vi "AG_PertApp.vi"() -> ()   [LabVIEW 2018]
doc: "The myRIO Project template acquires acceleration data from the onboard accelerometer and displays the changes of acceleration values in a waveform chart."
uses:
  <vilib>/Platform/TimedLoop/XDataNode/timing_clust.ctl
  <vilib>/Platform/TimedLoop/XDataNode/nitl_modes.ctl
  <vilib>/Platform/TimedLoop/XDataNode/wakeup.ctl
  <vilib>/Analysis/baseanly.llb/Mean (DBL).vi
  <vilib>/Analysis/1siggen.llb/Riffle Array (DBL).vi
  <vilib>/platform/TimedLoop/XDataNode/XDataNode.xnode
  <vilib>/Platform/TimedLoop/XDataNode/XDNodeRunTimeDep.lvlib
  <vilib>/Analysis/NI_AALBase.lvlib
  <vilib>/express/express signal manip/GetorSetDDTAttributes/Set DDT Attributes/Set DDT Properties.xnode
  <vilib>/express/express shared/transition.llb/Dynamic To Waveform Array.vi
  <vilib>/express/express signal manip/GetorSetDDTAttributes/Set DDT Attributes/SetT0.vi
  <vilib>/express/express shared/transition.llb/Waveform Array To Dynamic.vi
panel:
  in  "device name":tag="Dev1"
  in  "Developer Mode":bool
  out "Packet Array\nString":string
  out "Pert?":dbl
  in  "file path (use dialog)":path
  in  "Rest Steps\nCounter":bool
  in  "?":bool
  in  "Remote Port":u16=4000
  in  "IP Address":string="127.0.0.1"
  in  "Export Log Pathfile":path=path "test.xlsx" caption="Filename"
  in  "Perturbation Parameter\nArray Filepath":path=path "test.lvm" caption="Filename"
  in  "Perturbation \nSetting":enum32{"Predetermine", "Random", "Manual"}(radio)=enum."Manual"
  out "Step\nArray":dbl[](array[numeric])
  out "Perturbation\nArray":dbl[](array[numeric])
  in  "OK Button":bool
  out "Trial Number":dbl=1.0
  in  "Speed Parameter":enum32{"0.7 m/s Settings", "1.0 m/s Settings"}(radio)
  out "Packet Boolean":u32
  out "Packet \nArray":u8[][](array[numeric])
  out "Left vGRF (Filtered)":dynamicdata(graph)
  out "Step Counter":dbl
  in  "?":bool
  in  "GRF \nThreshold":dbl=30.0
  in  "Stance Fraction\nTrip":dbl=0.4
  out "Perturbation\nDelay Onset":dbl
  in  "LHS - Slip":bool
  in  "LHS Trip":bool
  in  "RHS - Slip":bool
  out "RHS?":bool
  out "TM Accel/\nDecel":dbl
  in  "RHS - Trip":bool
  out "HS Delay":dbl
  out "LHS?":bool
  in  "Slip/Trip \nTimer":dbl=0.2
  in  "Right Trip":bool
  in  "Left Trip":bool
  in  "Right Slip":bool
  in  "Left Slip":bool
  out "Right vGRF":dbl
  out "Left vGRF":dbl
  out "R-Stance\nMean":dbl format="%0.2f"
  out "LTO":dbl[](array[numeric])
  out "L-Stance Time":dbl[](array[numeric])
  out "LHS":dbl[](array[numeric])
  out "L-Stance\nMean":dbl format="%0.2f"
  out "R-Stance Time":dbl[](array[numeric])
  out "RTO":dbl[](array[numeric])
  out "RHS":dbl[](array[numeric])
  out "Elapsed Time (s)":dbl
  out "Right vGRF (Filtered)":dynamicdata(graph)
  in  "Stance Fraction\nSlip":dbl=0.4
  in  "Treadmill Control":bool
  in  "Treadmill Stop":bool
  in  "Belt Accel":dbl
  in  "Trip Speed":dbl
  in  "Slip Speed":dbl=2.0
  in  "Decelerate":dbl=10.0
  in  "Accelerate":dbl=10.0
  in  "Belt Speed":dbl(slide) min=0.0 step=0.1 scale=0.0..10.0
  out "TM Connection":errorcluster
  in  "Stop":bool
  # "Treadmill Control Protocol: READ FIRST\n\nBEFORE RUNNING VI\n1. Set \"Pertubration Parameters\" to either \"Predetermine\",\"Random\", or \"Manual\"\n\n1a. If set to \"Predetermine\", go into sub-VI and input all numbers into the \nPerturbation Array\" and \"Step Array\" in the \"Initialize\" part of the flat sequence\n\n2. Ensure all parameters are set to desired values. \n\n3. Optional: Input Filepath for text file \n\nSTART VI\n\n4. Press \"START\" on Treadmill Control Button. This will prevent the belt from accelerating more than 0.2 m/s^2. The treadmill will not start moving at this point\n\n5. Set Belt Speed to desired speed. \n\n5. Press \"Rest Step Counter\" to reset step counter once belt is up to speed\n\n6. DO NOT TURN OFF \"START\" TREADMILL CONTROL BUTTON UNTIL DESIRED SPEED IS MET! The treadmill will accelerate/decelerate at 10m/s^2 when the button is off\n\n7. Turn off \"START\"\"Treadmill Control Button once the desired speed is reached.\n\n8. Allow for a minimum of 5-steps per side to calculate average stance time for both feet\n\n9. Once average stance is calculated initiate a slip/trip my pressing Slip/Trip button for the corresponding side\n\n10. Allow for a minumum of 5-steps after perturbation to calculate average stance time again\n\n11. Continue steps 8-10 until all slips/trips have been performed.\n\n12. To slow the treadmill down, press the Treadmill \"STOP: button. This will decelerate the treadmill to 0 m/s at a rate of 0.2 m/s^2. \n\nIMPORTANT: If the belt speed needs to be changed after the initial speed is set, the \"START\" on theTreadmill Control Button must be enabled. If it is not enabled, the belt will accelerate at 10.0 m/s^2\n\nUse Left and Right Zero if needed"
  # "Perturbations"
  # "Perturabtion Paremeters"
  # "Developer Mode\n\nUse developer mode to test slipping protocol without vGRF data. \n\n1. Turn on \"Developer Mode\" button\n\n2. Press perturbation button\n\n3. Press corresponding developer button to emulate a heel strike"
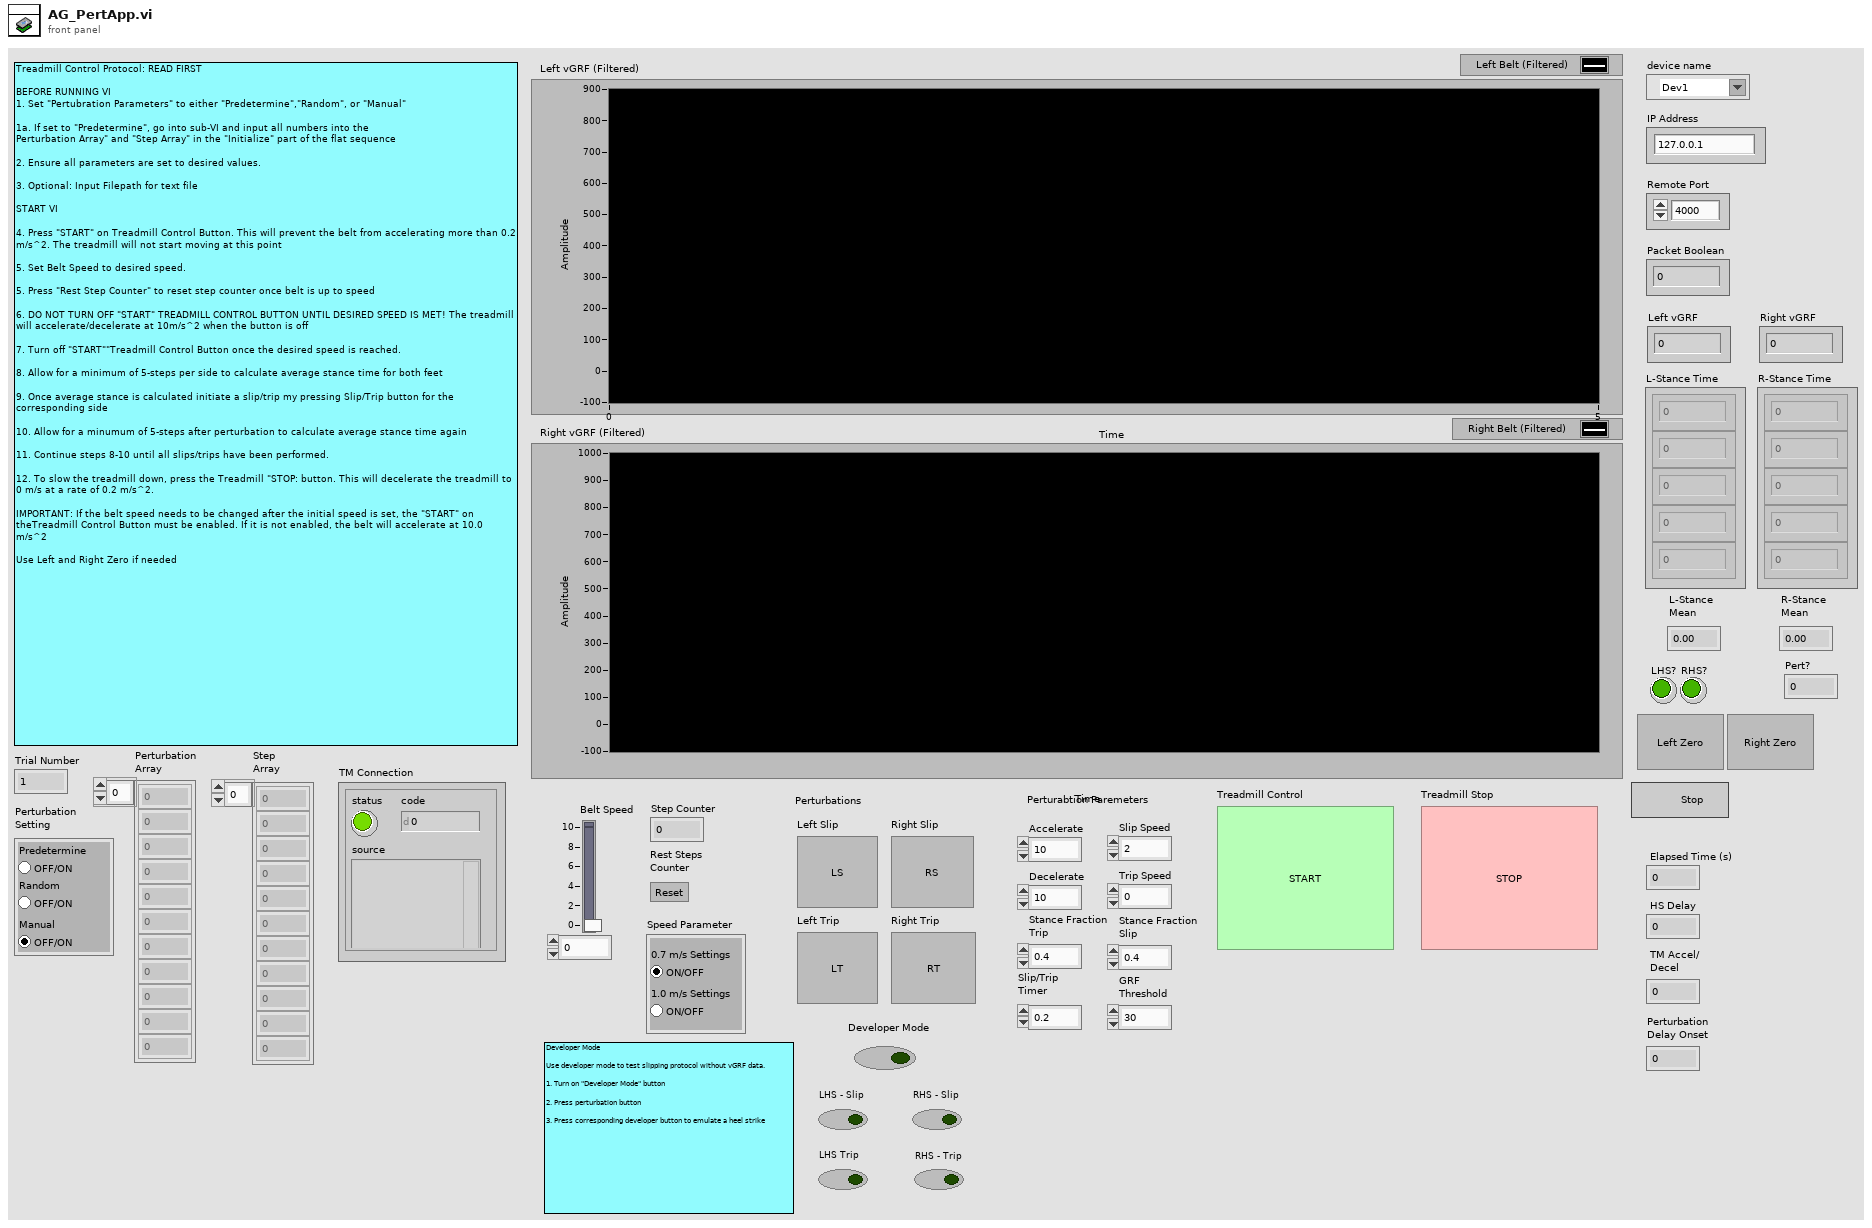
[diagram p1: front panel]
types:
  T1 = enum16{"open", "replace", "create", "open or create", "replace or create", "replace or create with confirmation"}
  T2 = enum16{"big-endian, network order", "native, host order", "little-endian"}
  T3 = typedef "XDNodeRunTimeDep.lvlib/timing_clust.ctl" = cluster{"Expected End [f-1]":u64, "Actual End [f-1]":u64, "Finished Late? [f-1]":bool, "Expected End [i-1]":u64, "Actual End [i-1]":u64, "Finished Late? [i-1]":bool, "Expected Start [i]":u64, "Actual Start [i]":u64, "Expected Start [f]":u64, "Actual Start [f]":u64, "Source Name":string, "Structure Name":string, "Period":i64, "Deadline":i64, "Offset":i64, "Start":i64, "Priority":i32, "Timeout":i32, "Mode":T4, "Wakeup Reason":T5, "Error":errorcluster, "Source Type":string, "Secondary Source Type":string, "Global End Time":u64, "Global Start Time":u64, "Frame Duration":u64, "Iteration Duration":u64, "Assigned CPU":i32, "I/O Scan Engine Mode":u32}
  T4 = typedef "XDNodeRunTimeDep.lvlib/nitl_modes.ctl" = enum32{"No Change", "Process missed periods, maintain original phase", "Discard missed periods, maintain original phase", "Process missed periods, ignore original phase", "Discard missed periods, ignore original phase"}
  T5 = typedef "XDNodeRunTimeDep.lvlib/wakeup.ctl" = enum32{"Normal", "Aborted", "Asynchronous wakeup", "Timing source error", "Timed loop error", "Timeout"}
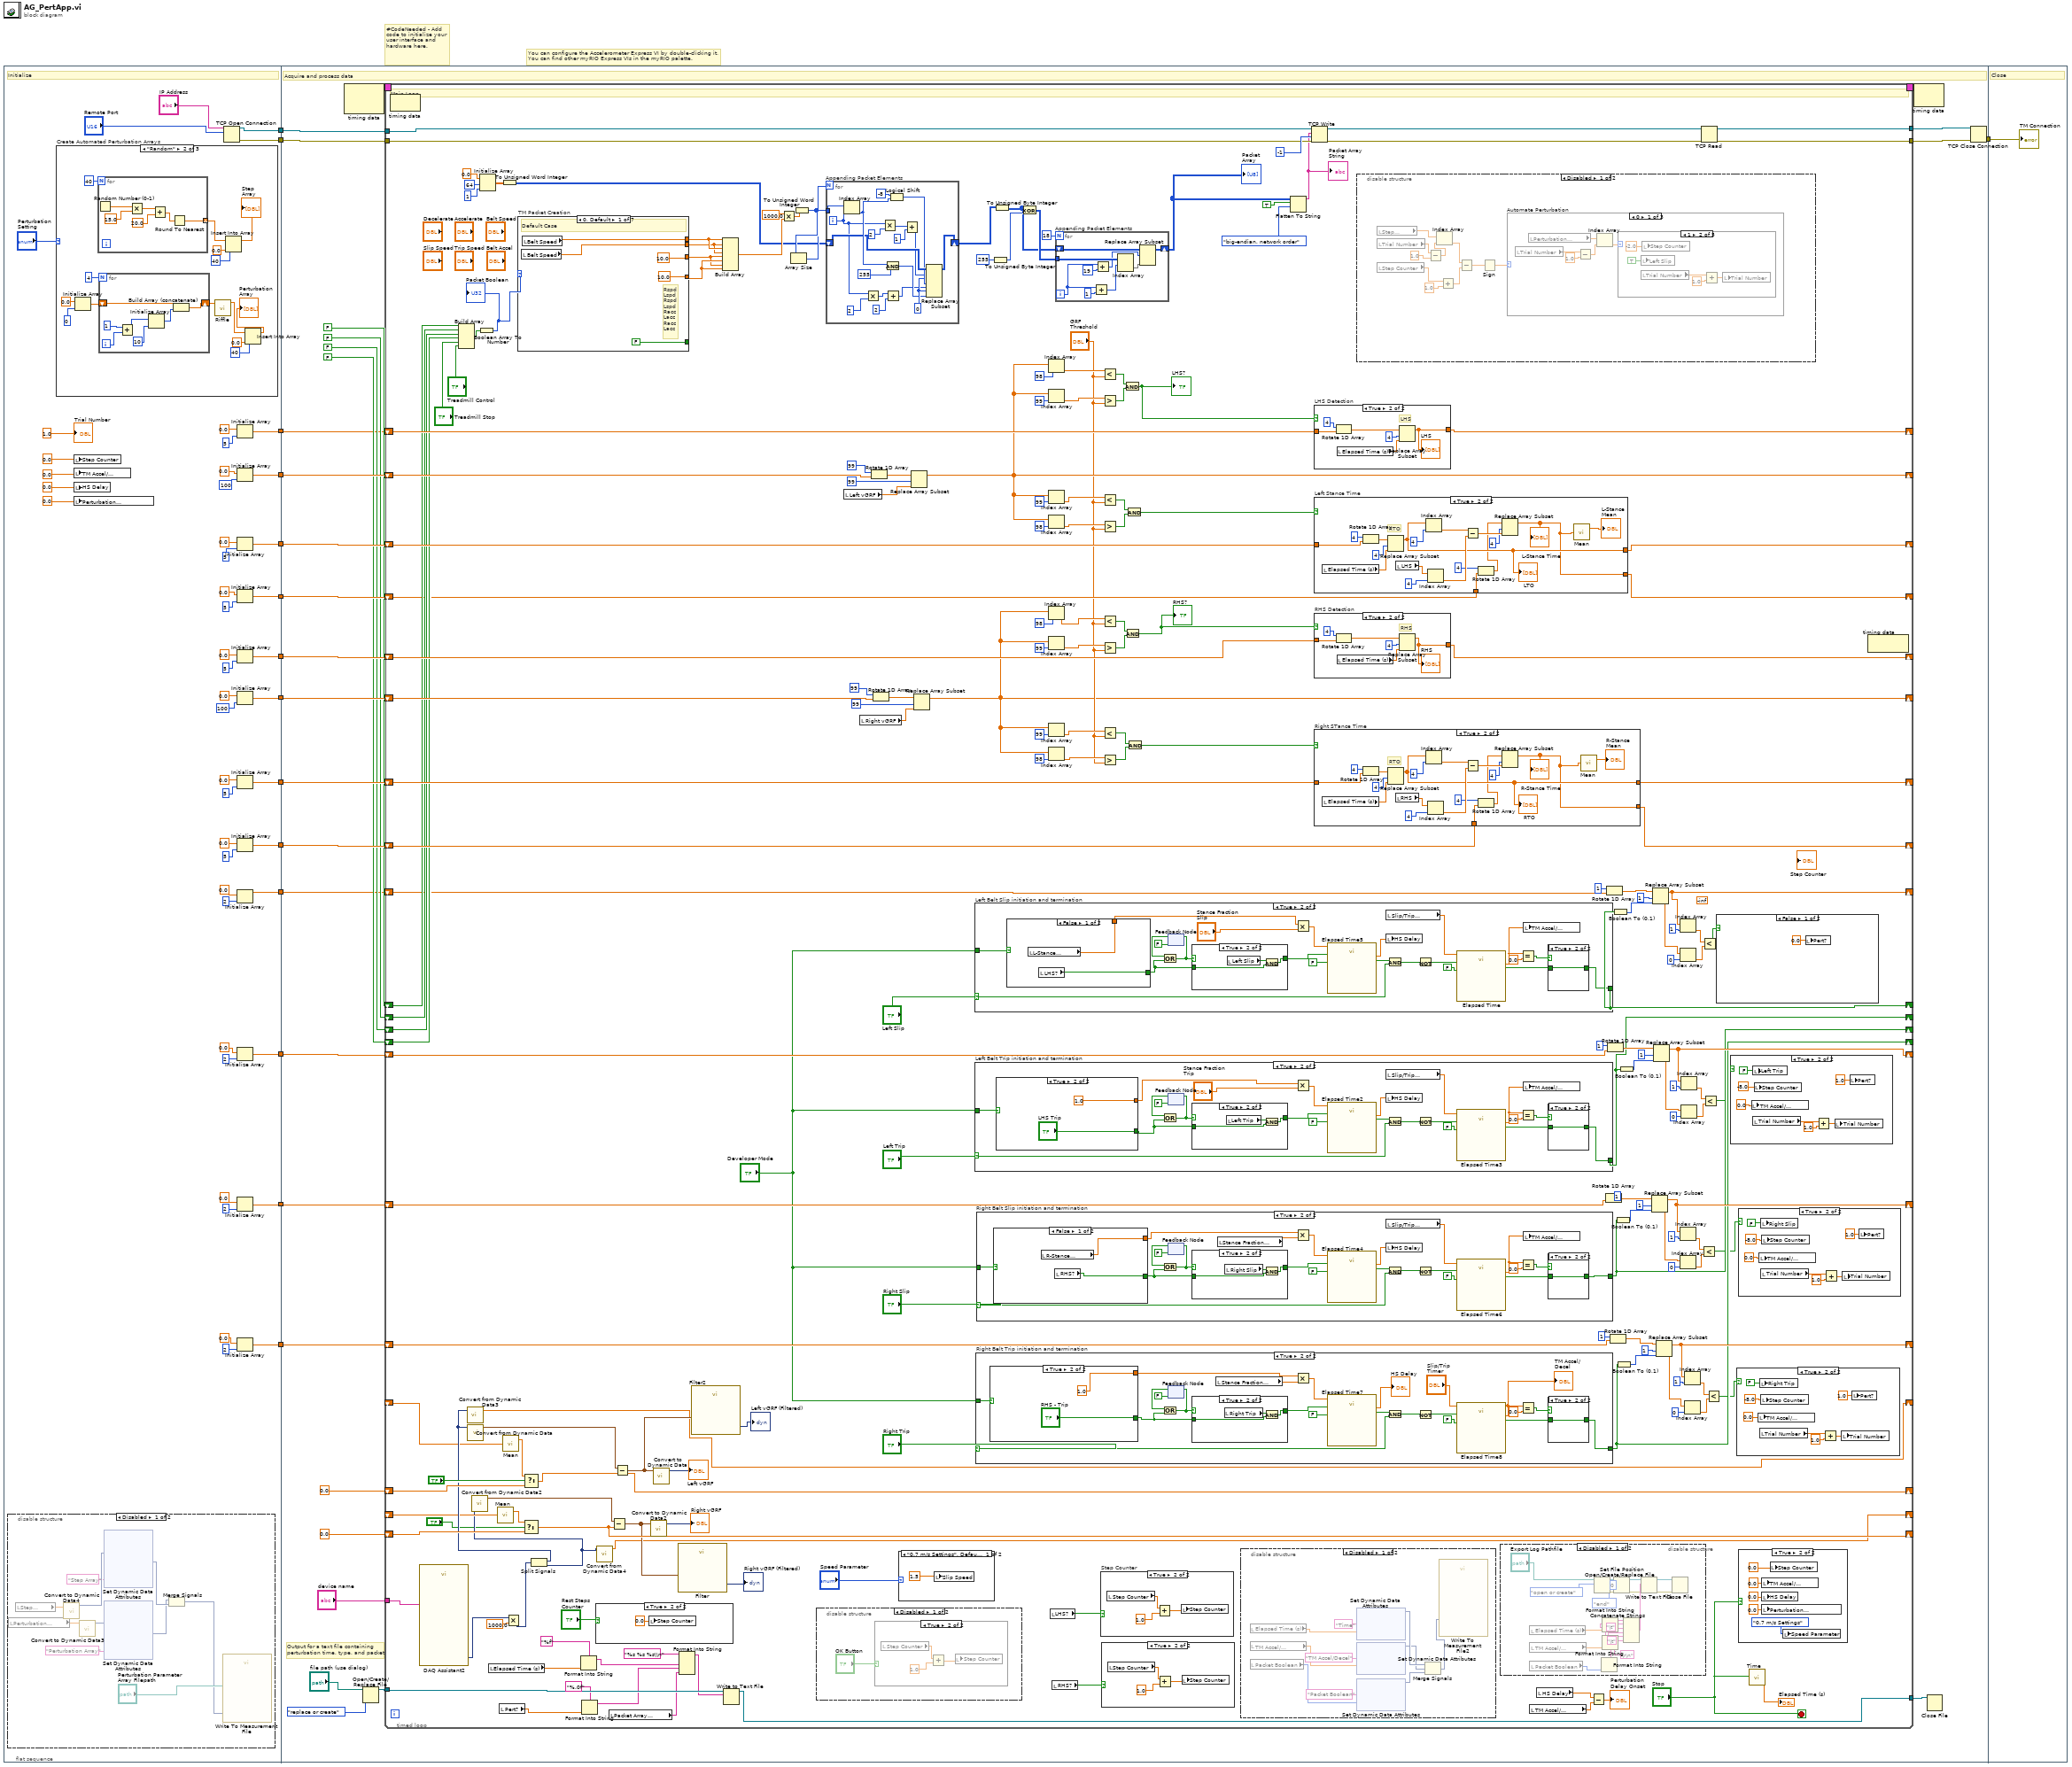
[diagram p0: block diagram]
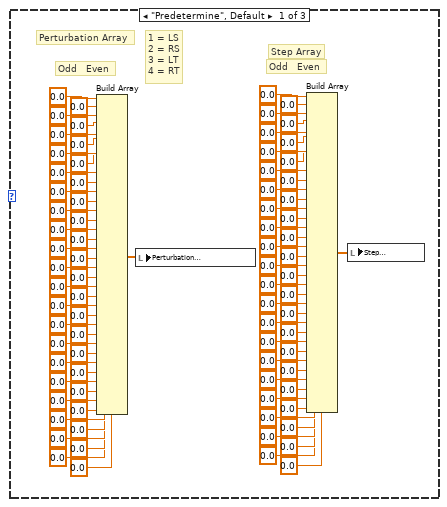
[diagram p3: hidden frame]
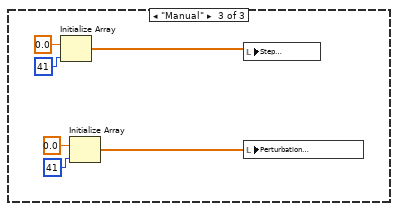
[diagram p4: hidden frame]
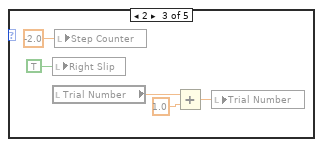
[diagram p7: hidden frame]
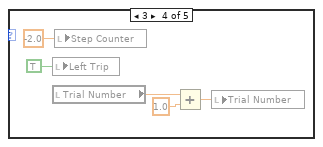
[diagram p8: hidden frame]
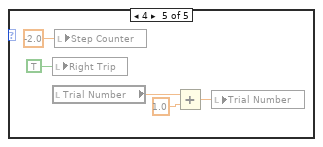
[diagram p9: hidden frame]
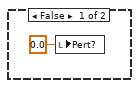
[diagram p17: hidden frame]
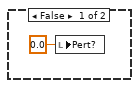
[diagram p18: hidden frame]
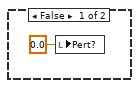
[diagram p19: hidden frame]
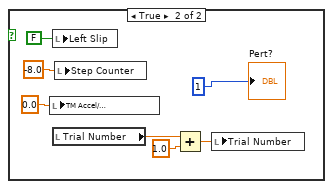
[diagram p20: hidden frame]
diagram:
  # "#CodeNeeded - Add code to initialize your user interface and hardware here."
  # "You can configure the Accelerometer Express VI by double-clicking it.\nYou can find other myRIO Express VIs in the myRIO palette."
  n1 = flat-sequence {
    tunnel: [w60] -> w15
    tunnel: [w59] -> w13
    tunnel: [w58] -> w12
    tunnel: [w53] -> w11
    tunnel: [w50] -> w10
    tunnel: [w44] -> w9
    tunnel: [w43] -> w8
    tunnel: [w40] -> w7
    tunnel: [w37] -> w6
    tunnel: [w34] -> w5
    tunnel: [w31] -> w4
    tunnel: [w28] -> w3
    tunnel: [w25] -> w2
    tunnel: [w22] -> w1
    tunnel: w15 -> [w244]
    tunnel: [w240] -> w14
    tunnel: w13 -> [w243]
    tunnel: w12 -> [w231]
    tunnel: w11 -> [w233]
    tunnel: w10 -> [w220]
    tunnel: w9 -> [w236]
    tunnel: w8 -> [w237]
    tunnel: w7 -> [w235]
    tunnel: w6 -> [w232]
    tunnel: w5 -> [w234]
    tunnel: w4 -> [w226]
    tunnel: w3 -> [w225]
    tunnel: w2 -> [w224]
    tunnel: w1 -> [w223]
    tunnel: w14 -> [w849]
    frame #0 {
      # "Initialize"
      n2 = disable-structure shown="Disabled" {
        frame Disabled {
          n3 = local read "Perturbation\nArray"() -> (w71:dbl[])
          n4 = local read "Step\nArray"() -> (w69:dbl[])
          n5 = call "Convert to Dynamic Data4"("Array"=w69) -> ("Dynamic Data Type"=w66:dynamicdata)  [unwired: 3 in]
          n6 = call "Convert to Dynamic Data3"("Array"=w71) -> ("Dynamic Data Type"=w67:dynamicdata)  [unwired: 3 in]
          n7 = xnode ("Set Dynamic Data Attributes")("Signals In"=w66, "Signal Name"="Step Array") -> ("Signals Out"=w65:dynamicdata)  [unwired: 2 in, 1 out]
          n8 = xnode ("Set Dynamic Data Attributes")("Signals In"=w67, "Signal Name"="Perturbation Array") -> ("Signals Out"=w64:dynamicdata)  [unwired: 2 in, 1 out]
          n9 = Merge Signals(w64, w65) -> (w68:dynamicdata)
          n10 = call "Write To Measurement File"("Signals"=w68, "Filename"="Perturbation Parameter\nArray Filepath") -> ()  [unwired: 15 in, 3 out]
        }
        frame Enabled {
        }
      }
      n11 = case "Create Automated Perturbation Arrays" shown="\"Random\"" "Perturbation \nSetting" {
        frame "Predetermine", Default {
          # "1 = LS\n2 = RS\n3 = LT\n4 = RT"
          # "Step Array"
          # "Perturbation Array"
          # "Odd   Even"
          # "Odd   Even"
          n12 = Build Array(0.0 ("element"), 0.0 ("element"), 0.0 ("element"), 0.0 ("element"), 0.0 ("element"), 0.0 ("element"), 0.0 ("element"), 0.0 ("element"), 0.0 ("element"), 0.0 ("element"), 0.0 ("element"), 0.0 ("element"), 0.0 ("element"), 0.0 ("element"), 0.0 ("element"), 0.0 ("element"), 0.0 ("element"), 0.0 ("element"), 0.0 ("element"), 0.0 ("element"), 0.0 ("element"), 0.0 ("element"), 0.0 ("element"), 0.0 ("element"), 0.0 ("element"), 0.0 ("element"), 0.0 ("element"), 0.0 ("element"), 0.0 ("element"), 0.0 ("element"), 0.0 ("element"), 0.0 ("element"), 0.0 ("element"), 0.0 ("element"), 0.0 ("element"), 0.0 ("element"), 0.0 ("element"), 0.0 ("element"), 0.0 ("element"), 0.0 ("element")) -> (w101:dbl[])
          n13 = local write "Perturbation\nArray"(w101) -> ()
          n14 = Build Array(0.0 ("element"), 0.0 ("element"), 0.0 ("element"), 0.0 ("element"), 0.0 ("element"), 0.0 ("element"), 0.0 ("element"), 0.0 ("element"), 0.0 ("element"), 0.0 ("element"), 0.0 ("element"), 0.0 ("element"), 0.0 ("element"), 0.0 ("element"), 0.0 ("element"), 0.0 ("element"), 0.0 ("element"), 0.0 ("element"), 0.0 ("element"), 0.0 ("element"), 0.0 ("element"), 0.0 ("element"), 0.0 ("element"), 0.0 ("element"), 0.0 ("element"), 0.0 ("element"), 0.0 ("element"), 0.0 ("element"), 0.0 ("element"), 0.0 ("element"), 0.0 ("element"), 0.0 ("element"), 0.0 ("element"), 0.0 ("element"), 0.0 ("element"), 0.0 ("element"), 0.0 ("element"), 0.0 ("element"), 0.0 ("element"), 0.0 ("element")) -> (w100:dbl[])
          n15 = local write "Step\nArray"(w100) -> ()
        }
        frame "Random" {
          n16 = Initialize Array(0.0 ("element"), 0 ("dimension size")) -> (w195:dbl[])
          n17 = for {
            N: 40 -> [_]
            tunnel: [w196] -> w189 mode=indexing
            n18 = Random Number (0-1)() -> (number: 0 to 1=w201:dbl)
            n19 = Multiply(x=w201, y=15.0) -> (x*y=w200:dbl)
            n20 = Add(x=w200, y=20.0) -> (x+y=w199:dbl)
            n21 = Round To Nearest(number=w199) -> (nearest integer value=w196:dbl)
          }
          n22 = for {
            N: 4 -> [_]
            shift-right: [w203] -> w191
            shift-left: w195 -> [w202]
            i -> [w207]
            n23 = Add(x=1, y=w207) -> (x+y=w206:i32)
            n24 = Initialize Array(w206, 10 ("dimension size")) -> (w204:i32[])
            n25 = Build Array (concatenate)(w202, w204) -> (w203:dbl[])
          }
          n26 = call-poly <vilib>:"Riffle.vi"("X"=w191) -> ("Riffled {X}"=w183:dbl[])  [unwired: 8 in, 2 out]
          n27 = Insert Into Array(array=w189, index=40, new element=0.0 ("new element/subarray")) -> (→"Step\nArray":dbl[])
          n28 = Insert Into Array(array=w183, index=40, new element=0.0 ("new element/subarray")) -> (→"Perturbation\nArray":dbl[])
        }
        frame "Manual" {
          n29 = Initialize Array(0.0 ("element"), 41 ("dimension size")) -> (w212:dbl[])
          n30 = Initialize Array(0.0 ("element"), 41 ("dimension size")) -> (w209:dbl[])
          n31 = local write "Step\nArray"(w212) -> ()
          n32 = local write "Perturbation\nArray"(w209) -> ()
        }
      }
      n33 = local write "Step Counter"(0.0 ("Step Counter")) -> ()
      n34 = local write "TM Accel/\nDecel"(0.0 ("Step Counter")) -> ()
      n35 = local write "HS Delay"(0.0 ("Step Counter")) -> ()
      n36 = local write "Perturbation\nDelay Onset"(0.0 ("Step Counter")) -> ()
      n37 = TCP Open Connection(address="IP Address", remote port or service name="Remote Port") -> (connection ID=w60:refnum<k5>, error out=w59:errorcluster)  [unwired: 3 in]
      n38 = Initialize Array(0.0 ("element"), 5 ("dimension size")) -> (w50:dbl[])
      n39 = Initialize Array(0.0 ("element"), 100 ("dimension size")) -> (w53:dbl[])
      n40 = Initialize Array(0.0 ("element"), 5 ("dimension size")) -> (w37:dbl[])
      n41 = Initialize Array(0.0 ("element"), 5 ("dimension size")) -> (w58:dbl[])
      n42 = Initialize Array(0.0 ("element"), 5 ("dimension size")) -> (w44:dbl[])
      n43 = Initialize Array(0.0 ("element"), 100 ("dimension size")) -> (w43:dbl[])
      n44 = Initialize Array(0.0 ("element"), 5 ("dimension size")) -> (w40:dbl[])
      n45 = Initialize Array(0.0 ("element"), 5 ("dimension size")) -> (w34:dbl[])
      n46 = Initialize Array(0.0 ("element"), 2 ("dimension size")) -> (w31:dbl[])
      n47 = Initialize Array(0.0 ("element"), 2 ("dimension size")) -> (w28:dbl[])
      n48 = Initialize Array(0.0 ("element"), 2 ("dimension size")) -> (w25:dbl[])
      n49 = Initialize Array(0.0 ("element"), 2 ("dimension size")) -> (w22:dbl[])
      "Trial Number" <- 1.0 ("Trial Number")
    }
    frame #1 {
      # "Output for a text file containing \nperturbation time, type, and packet"
      # "Acquire and process data"
      n50 = node-c288() -> (w239:T3)  [unwired: 2 in]
      n51 = Open/Create/Replace File(file path (use dialog)="file path (use dialog)", operation (0:open)=T1."replace or create") -> (refnum out=w217:refnum<file>)  [unwired: 4 in, 2 out]
      n52 = timed-loop {
        tunnel: w244 -> [w426]
        tunnel: w243 -> [w425]
        tunnel: [w433] -> w242
        tunnel: [w432] -> w241
        timing: w239 -> [_]
        timing-out: [_] -> w238
        shift-right: [w392] -> _
        shift-left: w236 -> [w390]
        shift-right: [w263] -> _
        shift-left: w237 -> [w391]
        shift-right: [w382] -> _
        shift-left: w235 -> [w383]
        shift-right: [w377] -> _
        shift-left: w234 -> [w378]
        shift-right: [w360] -> _
        shift-left: w233 -> [w366]
        shift-right: [w359] -> _
        shift-left: w220 -> [w361]
        shift-right: [w357] -> _
        shift-left: w232 -> [w358]
        shift-right: [w356] -> _
        shift-left: w231 -> [w350]
        shift-right: [w349] -> _
        shift-left: FALSE -> [w354]
        shift-right: [w328] -> _
        shift-left: FALSE -> [w353]
        shift-right: [w305] -> _
        shift-left: FALSE -> [w352]
        shift-right: [w304] -> _
        shift-left: FALSE -> [w351]
        shift-right: [w340] -> _
        shift-left: w226 -> [w347]
        shift-right: [w327] -> _
        shift-left: w225 -> [w329]
        shift-right: [w316] -> _
        shift-left: w224 -> [w317]
        shift-right: [w307] -> _
        shift-left: w223 -> [w306]
        shift-right: [w292] -> _
        shift-left: 0.0 -> [w294]
        shift-right: [w282] -> _
        shift-left: 0.0 -> [w291]
        shift-right: [w268] -> _
        shift-left: _ -> [w267]
        shift-right: [w264] -> _
        shift-left: _ -> [w266]
        tunnel: w217 -> [w257]
        tunnel: [w255] -> w216
        tunnel: "device name" -> [w245]
        stop <- "Stop" stop-if-true
        (unwired) -inf
        # "Main Loop"
        n53 = node-c288() -> ()  [unwired: 1 in, 1 out]
        n54 = call "DAQ Assistant2"("device name"=w245) -> ("data"=w261:dynamicdata)  [unwired: 15 in, 3 out]
        n55 = Build Array(w354, w353, w352, w351, "Treadmill Stop", "Treadmill Control") -> (w414:bool[])
        n56 = Boolean Array To Number(Boolean array=w414) -> (number=w412:u32)
        "Packet Boolean" <- w412
        n57 = Initialize Array(0.0 ("element"), 64 ("dimension size"), 1 ("dimension size")) -> (w408:dbl[][])
        n58 = local read "Elapsed Time (s)"() -> (w256:dbl)
        n59 = call-poly <vilib>:"Mean.vi"("X"=w266) -> ("mean"=w290:dbl)  [unwired: 1 out]
        n60 = local read "Pert?"() -> (w254:dbl)
        n61 = To Unsigned Word Integer(number=w408) -> (unsigned 16bit integer=w407:u16[][])
        n62 = call-poly <vilib>:"Mean.vi"("X"=w267) -> ("mean"=w293:dbl)  [unwired: 1 out]
        n63 = Multiply(x=w261, y=1000.0) -> (x*y=w355:dynamicdata)
        n64 = case "TM Packet Creation" shown="0, Default" w412 {
          tunnel: [FALSE w610 w615 w620 w625 FALSE FALSE] -> _
          tunnel: [w608 w614 w619 w624 w629 w630 w635] -> w298
          tunnel: [w609 w613 w618 w623 w628 w630 w635] -> w297
          tunnel: [10.0 w612 w617 w622 w627 w632 w634] -> w296
          tunnel: [10.0 w611 w616 w621 w626 w632 w634] -> w295
          frame 0, Default {
            # "Rspd\nLspd\nRspd\nLspd\nRacc\nLacc\nRacc\nLacc"
            # "Default Case"
            n65 = local read "Belt Speed"() -> (w609:dbl)
            n66 = local read "Belt Speed"() -> (w608:dbl)
          }
          frame 1 {
            w610 = FALSE
            # "Rspd\nLspd\nRspd\nLspd\nRacc\nLacc\nRacc\nLacc"
            # "Left Slip"
            n67 = local read "Belt Speed"() -> (w614:dbl)
            n68 = local read "Slip Speed"() -> (w613:dbl)
            n69 = local read "Accelerate"() -> (w611:dbl)
            n70 = local read "Accelerate"() -> (w612:dbl)
            n71 = local write "Treadmill Control"(w610) -> ()
          }
          frame 2 {
            w615 = FALSE
            # "Rspd\nLspd\nRspd\nLspd\nRacc\nLacc\nRacc\nLacc"
            # "Left Trip"
            n72 = local read "Trip Speed"() -> (w618:dbl)
            n73 = local read "Belt Speed"() -> (w619:dbl)
            n74 = local read "Decelerate"() -> (w616:dbl)
            n75 = local read "Decelerate"() -> (w617:dbl)
            n76 = local write "Treadmill Control"(w615) -> ()
          }
          frame 4 {
            w620 = FALSE
            # "Rspd\nLspd\nRspd\nLspd\nRacc\nLacc\nRacc\nLacc"
            # "Right Slip"
            n77 = local read "Belt Speed"() -> (w623:dbl)
            n78 = local read "Accelerate"() -> (w621:dbl)
            n79 = local read "Accelerate"() -> (w622:dbl)
            n80 = local read "Slip Speed"() -> (w624:dbl)
            n81 = local write "Treadmill Control"(w620) -> ()
          }
          frame 8 {
            w625 = FALSE
            # "Rspd\nLspd\nRspd\nLspd\nRacc\nLacc\nRacc\nLacc"
            # "Right Slip"
            n82 = local read "Trip Speed"() -> (w629:dbl)
            n83 = local read "Belt Speed"() -> (w628:dbl)
            n84 = local read "Decelerate"() -> (w626:dbl)
            n85 = local read "Decelerate"() -> (w627:dbl)
            n86 = local write "Treadmill Control"(w625) -> ()
          }
          frame 16, 48 {
            w632 = 0.2
            w630 = 0.0
            # "Stop Treadmill"
            n87 = local write "Belt Speed"(w630) -> ()
          }
          frame 15, 32 {
            w634 = 0.2 ("Decelerate")
            # "Start Treadmill"
            n88 = local read "Belt Speed"() -> (w635:dbl)
          }
        }
        n89 = Select(t=w290, s="?", f=w291) -> (s? t:f=w282:dbl)
        n90 = Select(t=w293, s="?", f=w294) -> (s? t:f=w292:dbl)
        n91 = Split Signals(w355) -> (w269:dynamicdata, w265:dynamicdata)  [unwired: 2 in]
        n92 = call "Convert from Dynamic Data3"("Dynamic Data Type"=w269) -> ("Array"=w268:dbl[])  [unwired: 3 in]
        n93 = call "Convert from Dynamic Data"("Dynamic Data Type"=w269) -> ("Array of Waveform"=w270:waveform(dbl)[])  [unwired: 3 in]
        n94 = call "Convert from Dynamic Data2"("Dynamic Data Type"=w265) -> ("Array of Waveform"=w289:waveform(dbl)[])  [unwired: 3 in]
        n95 = Format Into String(format string="%f", w256) -> (resulting string=w251:string)  [unwired: 2 in, 1 out]
        n96 = Format Into String(format string="%.0f", w254) -> (resulting string=w250:string)  [unwired: 2 in, 1 out]
        n97 = case shown="True" "Rest Steps\nCounter" {
          frame False {
          }
          frame True {
            n98 = local write "Step Counter"(0.0 ("Step Counter")) -> ()
          }
        }
        n99 = call "Convert from Dynamic Data4"("Dynamic Data Type"=w265) -> ("Array"=w264:dbl[])  [unwired: 3 in]
        n100 = local read "Packet Array\nString"() -> (w247:string)
        n101 = Subtract(x=w289, y=w282) -> (x-y=w272:waveform(dbl)[])
        n102 = Subtract(x=w270, y=w292) -> (x-y=w271:waveform(dbl)[])
        n103 = call "Convert to Dynamic Data2"("Array of Waveforms"=w272) -> ("Dynamic Data Type"=→"Right vGRF":dynamicdata)  [unwired: 3 in]
        n104 = call "Convert to Dynamic Data"("Array of Waveforms"=w271) -> ("Dynamic Data Type"=→"Left vGRF":dynamicdata)  [unwired: 3 in]
        n105 = call "Filter"("Signal"=w272) -> ("Filtered Signal"=→"Right vGRF (Filtered)":dynamicdata)  [unwired: 9 in, 1 out]
        n106 = Format Into String(format string="%s %s %s\\n", w251, w250, w247) -> (resulting string=w248:string)  [unwired: 2 in, 1 out]
        n107 = call "Filter2"("Signal"=w271) -> ("Filtered Signal"=→"Left vGRF (Filtered)":dynamicdata)  [unwired: 9 in, 1 out]
        n108 = Build Array(w298, w297, w298, w297, w295, w296, w295, w296) -> (w413:dbl[])
        n109 = Write to Text File(file (use dialog)=w257, text=w248) -> (refnum out=w255:refnum<file>)  [unwired: 2 in, 2 out]
        n110 = Multiply(x=1000.0 ("y"), y=w413) -> (x*y=w430:dbl[])
        n111 = To Unsigned Word Integer(number=w430) -> (unsigned 16bit integer=w424:u16[])
        n112 = Array Size(array=w424) -> (size(s)=w423:i32)
        n113 = disable-structure shown="Disabled" {
          frame Disabled {
            n114 = case shown="True" "OK Button" {
              frame False {
              }
              frame True {
                n115 = local read "Step Counter"() -> (w495:dbl)
                n116 = Add(x=w495, y=1.0) -> (x+y=w493:dbl)
                n117 = local write "Step Counter"(w493) -> ()
              }
            }
          }
          frame Enabled {
          }
        }
        n118 = for "Appending Packet Elements" {
          N: w423 -> [_]
          tunnel: w424 -> [w600]
          shift-right: [w597] -> w422
          shift-left: w407 -> [w596]
          i -> [w593]
          w589 = 0 ("disabled index (col)")
          n119 = Index Array(array=w600, index=w593) -> (element=w602:u16)
          n120 = Multiply(x=w593, y=2) -> (x*y=w590:i32)
          n121 = Multiply(x=w593, y=2) -> (x*y=w599:i32)
          n122 = And(x=w602, y=u16 255) -> (x .and. y?=w588:u16)
          n123 = Add(x=w590, y=2) -> (x+y=w587:i32)
          n124 = Logical Shift(y=i16 -8, x=w602) -> (x << y=w595:u16)
          n125 = Add(x=w599, y=1) -> (x+y=w594:i32)
          n126 = Replace Array Subset(array=w596, new element #1=w595, index (row) #1=w594, index (col) #1=w589, new element #2=w588, index (row) #2=w587, index (col) #2=w589) -> (w597:u16[][])
        }
        n127 = local read "Left vGRF"() -> (w380:dbl)
        n128 = local read "Right vGRF"() -> (w381:dbl)
        n129 = Rotate 1D Array(1:w366, 2:99 ("n")) -> (0:w416:dbl[])
        n130 = Rotate 1D Array(1:w391, 2:99 ("n")) -> (0:w399:dbl[])
        n131 = case shown="\"0.7 m/s Settings\", Default" "Speed Parameter" {
          frame "0.7 m/s Settings", Default {
            n132 = local write "Slip Speed"(1.5 ("Slip Speed")) -> ()
          }
          frame "1.0 m/s Settings" {
            n133 = local write "Slip Speed"(2.0 ("Slip Speed")) -> ()
          }
        }
        n134 = Replace Array Subset(array=w416, new element=w380, index=99) -> (w360:dbl[])
        n135 = Replace Array Subset(array=w399, new element=w381, index=99) -> (w263:dbl[])
        n136 = case "Left Belt Slip initiation and termination" shown="True" "Left Slip" {
          selector: "Left Slip" -> [w758 w769]
          tunnel: [w758 w780] -> w349
          tunnel: "Developer Mode" -> [_ w760]
          frame False {
          }
          frame True {
            n137 = case shown="False" w760 {
              tunnel: [w781 "LHS - Slip"] -> w761
              tunnel: [w782 1.0 ("x")] -> w759
              frame False {
                n138 = local read "L-Stance\nMean"() -> (w782:dbl)
                n139 = local read "LHS?"() -> (w781:bool)
              }
              frame True {
              }
            }
            n140 = feedback #1(FALSE) -> (w767:bool)
            n141 = Or(x=w767, y=w761) -> (x .or. y?=w770:bool)
            n142 = feedback-in #1(w770) -> ()
            n143 = case shown="True" w770 {
              selector: w770 -> [w785 _]
              tunnel: [w786 w787] -> w771
              tunnel: w761 -> [_ w788]
              frame False {
                n144 = Not(x=w785) -> (.not. x?=w786:bool)
              }
              frame True {
                n145 = local read "Left Slip"() -> (w789:bool)
                n146 = And(x=w789, y=w788) -> (x .and. y?=w787:bool)
              }
            }
            n147 = Multiply(x=w759, y="Stance Fraction\nSlip") -> (x*y=w766:dbl)
            n148 = call "Elapsed Time5"("Time Target (s)"=w766, "Reset"=w771, "Auto Reset"=FALSE) -> ("Elapsed Time (s)"=w763:dbl, "Time has Elapsed"=w768:bool)  [unwired: 9 in, 6 out]
            n149 = local read "Slip/Trip \nTimer"() -> (w764:dbl)
            n150 = local write "HS Delay"(w763) -> ()
            n151 = And(x=w768, y=w769) -> (x .and. y?=w773:bool)
            n152 = Not(x=w773) -> (.not. x?=w778:bool)
            n153 = call "Elapsed Time"("Time Target (s)"=w764, "Reset"=w778, "Auto Reset"=FALSE) -> ("Elapsed Time (s)"=w765:dbl, "Time has Elapsed"=w776:bool)  [unwired: 9 in, 6 out]
            n154 = Equal?(x=w765, y=0.0) -> (x = y?=w774:bool)
            n155 = local write "TM Accel/\nDecel"(w765) -> ()
            n156 = case shown="True" w774 {
              tunnel: [w791 w792] -> w780
              tunnel: w776 -> [w790 w792]
              frame False {
                n157 = Not(x=w790) -> (.not. x?=w791:bool)
              }
              frame True {
              }
            }
          }
        }
        n158 = case "Left Belt Trip initiation and termination" shown="True" "Left Trip" {
          selector: "Left Trip" -> [w723 w734]
          tunnel: [w723 w745] -> w328
          tunnel: "Developer Mode" -> [_ w724]
          frame False {
          }
          frame True {
            n159 = case shown="True" w724 {
              tunnel: [w746 "LHS Trip"] -> w726
              tunnel: [w747 1.0 ("x")] -> w725
              frame False {
                n160 = local read "L-Stance\nMean"() -> (w747:dbl)
                n161 = local read "LHS?"() -> (w746:bool)
              }
              frame True {
              }
            }
            n162 = feedback #2(FALSE) -> (w732:bool)
            n163 = Or(x=w732, y=w726) -> (x .or. y?=w735:bool)
            n164 = feedback-in #2(w735) -> ()
            n165 = case shown="True" w735 {
              selector: w735 -> [w750 _]
              tunnel: [w751 w752] -> w736
              tunnel: w726 -> [_ w753]
              frame False {
                n166 = Not(x=w750) -> (.not. x?=w751:bool)
              }
              frame True {
                n167 = local read "Left Trip"() -> (w754:bool)
                n168 = And(x=w754, y=w753) -> (x .and. y?=w752:bool)
              }
            }
            n169 = Multiply(x=w725, y="Stance Fraction\nTrip") -> (x*y=w731:dbl)
            n170 = call "Elapsed Time2"("Time Target (s)"=w731, "Reset"=w736, "Auto Reset"=FALSE) -> ("Elapsed Time (s)"=w728:dbl, "Time has Elapsed"=w733:bool)  [unwired: 9 in, 6 out]
            n171 = local read "Slip/Trip \nTimer"() -> (w729:dbl)
            n172 = local write "HS Delay"(w728) -> ()
            n173 = And(x=w733, y=w734) -> (x .and. y?=w738:bool)
            n174 = Not(x=w738) -> (.not. x?=w743:bool)
            n175 = call "Elapsed Time3"("Time Target (s)"=w729, "Reset"=w743, "Auto Reset"=FALSE) -> ("Elapsed Time (s)"=w730:dbl, "Time has Elapsed"=w741:bool)  [unwired: 9 in, 6 out]
            n176 = Equal?(x=w730, y=0.0) -> (x = y?=w739:bool)
            n177 = local write "TM Accel/\nDecel"(w730) -> ()
            n178 = case shown="True" w739 {
              tunnel: [w756 w757] -> w745
              tunnel: w741 -> [w755 w757]
              frame False {
                n179 = Not(x=w755) -> (.not. x?=w756:bool)
              }
              frame True {
              }
            }
          }
        }
        n180 = case "Right Belt Trip initiation and termination" shown="True" "Right Trip" {
          selector: "Right Trip" -> [w653 w664]
          tunnel: [w653 w675] -> w304
          tunnel: "Developer Mode" -> [_ w654]
          frame False {
          }
          frame True {
            n181 = case shown="True" w654 {
              tunnel: [w676 "RHS - Trip"] -> w656
              tunnel: [w677 1.0 ("x")] -> w655
              frame False {
                n182 = local read "R-Stance\nMean"() -> (w677:dbl)
                n183 = local read "RHS?"() -> (w676:bool)
              }
              frame True {
              }
            }
            n184 = feedback #3(FALSE) -> (w662:bool)
            n185 = Or(x=w662, y=w656) -> (x .or. y?=w665:bool)
            n186 = feedback-in #3(w665) -> ()
            n187 = case shown="True" w665 {
              selector: w665 -> [w680 _]
              tunnel: [w681 w682] -> w666
              tunnel: w656 -> [_ w683]
              frame False {
                n188 = Not(x=w680) -> (.not. x?=w681:bool)
              }
              frame True {
                n189 = local read "Right Trip"() -> (w684:bool)
                n190 = And(x=w684, y=w683) -> (x .and. y?=w682:bool)
              }
            }
            n191 = local read "Stance Fraction\nTrip"() -> (w657:dbl)
            n192 = Multiply(x=w655, y=w657) -> (x*y=w661:dbl)
            n193 = call "Elapsed Time7"("Time Target (s)"=w661, "Reset"=w666, "Auto Reset"=FALSE) -> ("Elapsed Time (s)"=→"HS Delay":dbl, "Time has Elapsed"=w663:bool)  [unwired: 9 in, 6 out]
            n194 = And(x=w663, y=w664) -> (x .and. y?=w668:bool)
            n195 = Not(x=w668) -> (.not. x?=w673:bool)
            n196 = call "Elapsed Time8"("Time Target (s)"="Slip/Trip \nTimer", "Reset"=w673, "Auto Reset"=FALSE) -> ("Elapsed Time (s)"=w658:dbl, "Time has Elapsed"=w671:bool)  [unwired: 9 in, 6 out]
            "TM Accel/\nDecel" <- w658
            n197 = Equal?(x=w658, y=0.0) -> (x = y?=w669:bool)
            n198 = case shown="True" w669 {
              tunnel: [w686 w687] -> w675
              tunnel: w671 -> [w685 w687]
              frame False {
                n199 = Not(x=w685) -> (.not. x?=w686:bool)
              }
              frame True {
              }
            }
          }
        }
        n200 = case "Right Belt Slip initiation and termination" shown="True" "Right Slip" {
          selector: "Right Slip" -> [w688 w699]
          tunnel: [w688 w710] -> w305
          tunnel: "Developer Mode" -> [_ w689]
          frame False {
          }
          frame True {
            n201 = case shown="False" w689 {
              tunnel: [w711 "RHS - Slip"] -> w691
              tunnel: [w712 1.0 ("x")] -> w690
              frame False {
                n202 = local read "R-Stance\nMean"() -> (w712:dbl)
                n203 = local read "RHS?"() -> (w711:bool)
              }
              frame True {
              }
            }
            n204 = feedback #4(FALSE) -> (w697:bool)
            n205 = Or(x=w697, y=w691) -> (x .or. y?=w700:bool)
            n206 = feedback-in #4(w700) -> ()
            n207 = case shown="True" w700 {
              selector: w700 -> [w715 _]
              tunnel: [w716 w717] -> w701
              tunnel: w691 -> [_ w718]
              frame False {
                n208 = Not(x=w715) -> (.not. x?=w716:bool)
              }
              frame True {
                n209 = local read "Right Slip"() -> (w719:bool)
                n210 = And(x=w719, y=w718) -> (x .and. y?=w717:bool)
              }
            }
            n211 = local read "Stance Fraction\nSlip"() -> (w692:dbl)
            n212 = Multiply(x=w690, y=w692) -> (x*y=w696:dbl)
            n213 = call "Elapsed Time4"("Time Target (s)"=w696, "Reset"=w701, "Auto Reset"=FALSE) -> ("Elapsed Time (s)"=w693:dbl, "Time has Elapsed"=w698:bool)  [unwired: 9 in, 6 out]
            n214 = local read "Slip/Trip \nTimer"() -> (w694:dbl)
            n215 = local write "HS Delay"(w693) -> ()
            n216 = And(x=w698, y=w699) -> (x .and. y?=w703:bool)
            n217 = Not(x=w703) -> (.not. x?=w708:bool)
            n218 = call "Elapsed Time6"("Time Target (s)"=w694, "Reset"=w708, "Auto Reset"=FALSE) -> ("Elapsed Time (s)"=w695:dbl, "Time has Elapsed"=w706:bool)  [unwired: 9 in, 6 out]
            n219 = Equal?(x=w695, y=0.0) -> (x = y?=w704:bool)
            n220 = local write "TM Accel/\nDecel"(w695) -> ()
            n221 = case shown="True" w704 {
              tunnel: [w721 w722] -> w710
              tunnel: w706 -> [w720 w722]
              frame False {
                n222 = Not(x=w720) -> (.not. x?=w721:bool)
              }
              frame True {
              }
            }
          }
        }
        n223 = To Unsigned Byte Integer(number=u8 255) -> (unsigned 8bit integer=w428:u8)
        n224 = To Unsigned Byte Integer(number=w422) -> (unsigned 8bit integer=w419:u8[][])
        n225 = Exclusive Or(1:w428, 2:w419) -> (0:w420:u8[][])
        n226 = Index Array(array=w360, index=98) -> (element=w362:dbl)
        n227 = Index Array(array=w360, index=99) -> (element=w363:dbl)
        n228 = Index Array(array=w360, index=99) -> (element=w364:dbl)
        n229 = Index Array(array=w360, index=98) -> (element=w365:dbl)
        n230 = Index Array(array=w263, index=98) -> (element=w395:dbl)
        n231 = Index Array(array=w263, index=99) -> (element=w393:dbl)
        n232 = Index Array(array=w263, index=99) -> (element=w385:dbl)
        n233 = Index Array(array=w263, index=98) -> (element=w384:dbl)
        n234 = local read "LHS?"() -> (w286:bool)
        n235 = local read "RHS?"() -> (w285:bool)
        n236 = for "Appending Packet Elements" {
          N: 18 -> [_]
          shift-right: [w644] -> w418
          shift-left: w419 -> [w643]
          tunnel: w420 -> [w641]
          i -> [w639]
          n237 = Add(x=w639, y=1) -> (x+y=w640:i32)
          n238 = Add(x=w639, y=19) -> (x+y=w637:i32)
          n239 = Index Array(array=w641, index (row)=w640) -> (element=w642:u8[])  [unwired: 1 in]
          n240 = Replace Array Subset(array=w643, new element=w642, index (row)=w637) -> (w644:u8[][])  [unwired: 1 in]
        }
        "Packet \nArray" <- w418
        n241 = case "Step Counter" shown="True" w286 {
          frame False {
          }
          frame True {
            n242 = local read "Step Counter"() -> (w652:dbl)
            n243 = Add(x=w652, y=1.0) -> (x+y=w650:dbl)
            n244 = local write "Step Counter"(w650) -> ()
          }
        }
        n245 = case shown="True" w285 {
          frame False {
          }
          frame True {
            n246 = local read "Step Counter"() -> (w649:dbl)
            n247 = Add(x=w649, y=1.0) -> (x+y=w647:dbl)
            n248 = local write "Step Counter"(w647) -> ()
          }
        }
        n249 = Less?(x=w362, y="GRF \nThreshold") -> (x < y?=w376:bool)
        n250 = Greater?(x=w363, y="GRF \nThreshold") -> (0:w375:bool)
        n251 = Less?(x=w364, y="GRF \nThreshold") -> (x < y?=w369:bool)
        n252 = Greater?(x=w365, y="GRF \nThreshold") -> (0:w368:bool)
        n253 = Less?(x=w395, y="GRF \nThreshold") -> (x < y?=w402:bool)
        n254 = Greater?(x=w393, y="GRF \nThreshold") -> (0:w401:bool)
        n255 = Less?(x=w385, y="GRF \nThreshold") -> (x < y?=w387:bool)
        n256 = Greater?(x=w384, y="GRF \nThreshold") -> (0:w386:bool)
        n257 = And(x=w376, y=w375) -> (x .and. y?=w372:bool)
        "LHS?" <- w372
        n258 = And(x=w402, y=w401) -> (x .and. y?=w394:bool)
        "RHS?" <- w394
        n259 = And(x=w369, y=w368) -> (x .and. y?=w367:bool)
        n260 = And(x=w387, y=w386) -> (x .and. y?=w379:bool)
        n261 = disable-structure shown="Disabled" {
          frame Disabled {
            n262 = local read "Elapsed Time (s)"() -> (w505:dbl)
            n263 = local read "TM Accel/\nDecel"() -> (w504:dbl)
            n264 = local read "Packet Boolean"() -> (w503:u32)
            n265 = xnode ("Set Dynamic Data Attributes")("Signals In"=w505, "Signal Name"="Time") -> ("Signals Out"=w502:dynamicdata)  [unwired: 2 in, 1 out]
            n266 = xnode ("Set Dynamic Data Attributes")("Signals In"=w504, "Signal Name"="TM Accel/Decel") -> ("Signals Out"=w501:dynamicdata)  [unwired: 2 in, 1 out]
            n267 = xnode ("Set Dynamic Data Attributes")("Signals In"=w503, "Signal Name"="Packet Boolean") -> ("Signals Out"=w500:dynamicdata)  [unwired: 2 in, 1 out]
            n268 = Merge Signals(w502, w501, w500) -> (w496:dynamicdata)
            n269 = call "Write To Measurement File2"("Signals"=w496) -> ()  [unwired: 16 in, 3 out]
          }
          frame Enabled {
          }
        }
        n270 = Flatten To String(anything=w418, prepend array or string size? (T)=TRUE, byte order (0:big-endian, network order)=T2."big-endian, network order") -> (data string=w284:string)  [unwired: 1 in, 2 out]
        "Packet Array\nString" <- w284
        n271 = TCP Write(connection ID=w426, data in=w284, error in (no error)=w425, 9:-1 ("timeout ms (25000)")) -> (connection ID out=w435:refnum<k5>, error out=w434:errorcluster)  [unwired: 1 out]
        n272 = case "LHS Detection" shown="True" w372 {
          tunnel: [w813 w815] -> w359
          tunnel: w361 -> [w813 w814]
          frame False {
          }
          frame True {
            # "LHS"
            n273 = Rotate 1D Array(1:w814, 2:4 ("n")) -> (0:w817:dbl[])
            n274 = local read "Elapsed Time (s)"() -> (w816:dbl)
            n275 = Replace Array Subset(array=w817, new element=w816, index=4) -> (w815:dbl[])
            "LHS" <- w815
          }
        }
        n276 = case "Left Stance Time" shown="True" w367 {
          tunnel: [w793 w804] -> w357
          tunnel: [w794 w796] -> w356
          tunnel: w358 -> [w793 w798]
          tunnel: w350 -> [w794 w797]
          frame False {
          }
          frame True {
            # "RTO"
            n277 = local read "Elapsed Time (s)"() -> (w809:dbl)
            n278 = Rotate 1D Array(1:w798, 2:4 ("n")) -> (0:w812:dbl[])
            n279 = Replace Array Subset(array=w812, new element=w809, index=4) -> (w804:dbl[])
            "LTO" <- w804
            n280 = local read "LHS"() -> (w803:dbl[])
            n281 = Index Array(array=w804, index=4) -> (element=w808:dbl)
            n282 = Index Array(array=w803, index=4) -> (element=w807:dbl)
            n283 = Subtract(x=w808, y=w807) -> (x-y=w802:dbl)
            n284 = Rotate 1D Array(1:w797, 2:4 ("index")) -> (0:w799:dbl[])
            n285 = Replace Array Subset(array=w799, new element=w802, index=4) -> (w796:dbl[])
            "L-Stance Time" <- w796
            n286 = call-poly <vilib>:"Mean.vi"("X"=w796) -> ("mean"=→"L-Stance\nMean":dbl)  [unwired: 1 out]
          }
        }
        n287 = case "RHS Detection" shown="True" w394 {
          tunnel: [w840 w841] -> w392
          tunnel: w390 -> [w840 w843]
          frame False {
          }
          frame True {
            # "RHS"
            n288 = Rotate 1D Array(1:w843, 2:4 ("n")) -> (0:w844:dbl[])
            n289 = local read "Elapsed Time (s)"() -> (w842:dbl)
            n290 = Replace Array Subset(array=w844, new element=w842, index=4) -> (w841:dbl[])
            "RHS" <- w841
          }
        }
        n291 = case "Right STance Time" shown="True" w379 {
          tunnel: w383 -> [w821 w836]
          tunnel: [w821 w830] -> w382
          tunnel: w378 -> [w820 w826]
          tunnel: [w820 w823] -> w377
          frame False {
          }
          frame True {
            # "RTO"
            n292 = local read "Elapsed Time (s)"() -> (w835:dbl)
            n293 = Rotate 1D Array(1:w836, 2:4 ("n")) -> (0:w839:dbl[])
            n294 = Replace Array Subset(array=w839, new element=w835, index=4) -> (w830:dbl[])
            "RTO" <- w830
            n295 = local read "RHS"() -> (w829:dbl[])
            n296 = Index Array(array=w830, index=4) -> (element=w834:dbl)
            n297 = Index Array(array=w829, index=4) -> (element=w833:dbl)
            n298 = Subtract(x=w834, y=w833) -> (x-y=w828:dbl)
            n299 = Rotate 1D Array(1:w826, 2:4 ("index")) -> (0:w824:dbl[])
            n300 = Replace Array Subset(array=w824, new element=w828, index=4) -> (w823:dbl[])
            "R-Stance Time" <- w823
            n301 = call-poly <vilib>:"Mean.vi"("X"=w823) -> ("mean"=→"R-Stance\nMean":dbl)  [unwired: 1 out]
          }
        }
        n302 = disable-structure shown="Disabled" {
          frame Disabled {
            n303 = local read "Step\nArray"() -> (w446:dbl[])
            n304 = local read "Trial Number"() -> (w439:dbl)
            n305 = local read "Step Counter"() -> (w442:dbl)
            n306 = Subtract(x=w439, y=1.0) -> (x-y=w438:dbl)
            n307 = Index Array(array=w446, index=w438) -> (element=w445:dbl)
            n308 = Add(x=w442, y=1.0) -> (x+y=w440:dbl)
            n309 = Subtract(x=w445, y=w440) -> (x-y=w444:dbl)
            n310 = Sign(1:w444) -> (0:w443:dbl)
            n311 = case "Automate Perturbation" shown="0" w443 {
              frame 0 {
                n312 = local read "Trial Number"() -> (w448:dbl)
                n313 = local read "Perturbation\nArray"() -> (w451:dbl[])
                n314 = Subtract(x=w448, y=1.0) -> (x-y=w447:dbl)
                n315 = Index Array(array=w451, index=w447) -> (element=w450:dbl)
                n316 = case shown="1" w450 {
                  frame 0, Default {
                  }
                  frame 1 {
                    n317 = local write "Left Slip"(TRUE) -> ()
                    n318 = local read "Trial Number"() -> (w455:dbl)
                    n319 = local write "Step Counter"(-2.0 ("Step Counter")) -> ()
                    n320 = Add(x=w455, y=1.0) -> (x+y=w453:dbl)
                    n321 = local write "Trial Number"(w453) -> ()
                  }
                  frame 2 {
                    n322 = local write "Right Slip"(TRUE) -> ()
                    n323 = local read "Trial Number"() -> (w460:dbl)
                    n324 = local write "Step Counter"(-2.0 ("Step Counter")) -> ()
                    n325 = Add(x=w460, y=1.0) -> (x+y=w458:dbl)
                    n326 = local write "Trial Number"(w458) -> ()
                  }
                  frame 3 {
                    n327 = local write "Left Trip"(TRUE) -> ()
                    n328 = local read "Trial Number"() -> (w465:dbl)
                    n329 = local write "Step Counter"(-2.0 ("Step Counter")) -> ()
                    n330 = Add(x=w465, y=1.0) -> (x+y=w463:dbl)
                    n331 = local write "Trial Number"(w463) -> ()
                  }
                  frame 4 {
                    n332 = local write "Right Trip"(TRUE) -> ()
                    n333 = local read "Trial Number"() -> (w470:dbl)
                    n334 = local write "Step Counter"(-2.0 ("Step Counter")) -> ()
                    n335 = Add(x=w470, y=1.0) -> (x+y=w468:dbl)
                    n336 = local write "Trial Number"(w468) -> ()
                  }
                }
              }
              frame 1, Default {
              }
              frame -1 {
              }
            }
          }
          frame Enabled {
          }
        }
        n337 = disable-structure shown="Disabled" {
          frame Disabled {
            n338 = local read "Elapsed Time (s)"() -> (w485:dbl)
            n339 = local read "TM Accel/\nDecel"() -> (w482:dbl)
            n340 = local read "Packet Boolean"() -> (w474:u32)
            n341 = Open/Create/Replace File(file path (use dialog)="Export Log Pathfile", operation (0:open)=T1."open or create") -> (refnum out=w477:refnum<file>, error out=w481:errorcluster)  [unwired: 4 in, 1 out]
            n342 = Format Into String(w474) -> (resulting string=w473:string)  [unwired: 3 in, 1 out]
            n343 = Format Into String(w485) -> (resulting string=w486:string)  [unwired: 3 in, 1 out]
            n344 = Format Into String(w482) -> (resulting string=w489:string)  [unwired: 3 in, 1 out]
            n345 = Set File Position(offset (in bytes) (0)=i64 0, refnum=w477, from (0:start)=enum16{"start", "end", "current"}."end", error in=w481) -> (refnum out=w483:refnum<file>, error out=w484:errorcluster)
            n346 = Concatenate Strings(w486, "\t", w489, "\t", w473, "\r\n") -> (w488:string)
            n347 = Write to Text File(file (use dialog)=w483, text=w488, error in=w484) -> (refnum out=w490:refnum<file>, error out=w491:errorcluster)  [unwired: 1 in, 1 out]
            n348 = Close File(refnum=w490, error in=w491) -> ()  [unwired: 2 out]
          }
          frame Enabled {
          }
        }
        n349 = local read "TM Accel/\nDecel"() -> (w302:dbl)
        n350 = local read "HS Delay"() -> (w303:dbl)
        n351 = Subtract(x=w303, y=w302) -> (x-y=→"Perturbation\nDelay Onset":dbl)
        n352 = Rotate 1D Array(1:w317, 2:1 ("n")) -> (0:w323:dbl[])
        n353 = Rotate 1D Array(1:w347, 2:1 ("n")) -> (0:w345:dbl[])
        n354 = Rotate 1D Array(1:w329, 2:1 ("n")) -> (0:w335:dbl[])
        n355 = Rotate 1D Array(1:w306, 2:1 ("n")) -> (0:w313:dbl[])
        n356 = Boolean To (0,1)(Boolean=w349) -> (0, 1=w348:i16)
        n357 = Boolean To (0,1)(Boolean=w305) -> (0, 1=w325:i16)
        n358 = Boolean To (0,1)(Boolean=w304) -> (0, 1=w315:i16)
        n359 = Boolean To (0,1)(Boolean=w328) -> (0, 1=w337:i16)
        n360 = Replace Array Subset(array=w323, new element=w325, index=1) -> (w316:dbl[])
        n361 = Replace Array Subset(array=w345, new element=w348, index=1) -> (w340:dbl[])
        n362 = Replace Array Subset(array=w335, new element=w337, index=1) -> (w327:dbl[])
        n363 = Replace Array Subset(array=w313, new element=w315, index=1) -> (w307:dbl[])
        n364 = Index Array(array=w316, index=1) -> (element=w320:dbl)
        n365 = Index Array(array=w316, index=0) -> (element=w319:dbl)
        n366 = Index Array(array=w340, index=1) -> (element=w342:dbl)
        n367 = Index Array(array=w340, index=0) -> (element=w341:dbl)
        n368 = Index Array(array=w327, index=1) -> (element=w332:dbl)
        n369 = Index Array(array=w327, index=0) -> (element=w331:dbl)
        n370 = Index Array(array=w307, index=1) -> (element=w310:dbl)
        n371 = Index Array(array=w307, index=0) -> (element=w309:dbl)
        n372 = TCP Read(connection ID=w435, error in (no error)=w434) -> (connection ID out=w432:refnum<k5>, error out=w433:errorcluster)  [unwired: 3 in, 1 out]
        n373 = Less?(x=w320, y=w319) -> (x < y?=w279:bool)
        n374 = Less?(x=w342, y=w341) -> (x < y?=w277:bool)
        n375 = Less?(x=w332, y=w331) -> (x < y?=w278:bool)
        n376 = Less?(x=w310, y=w309) -> (x < y?=w280:bool)
        n377 = case shown="False" w277 {
          frame False {
            n378 = local write "Pert?"(0.0 ("Pert?")) -> ()
          }
          frame True {
            n379 = local write "TM Accel/\nDecel"(0.0 ("Step Counter")) -> ()
            n380 = local write "Left Slip"(FALSE) -> ()
            n381 = local read "Trial Number"() -> (w578:dbl)
            n382 = local write "Step Counter"(-8.0 ("Step Counter")) -> ()
            n383 = Add(x=w578, y=1.0) -> (x+y=w576:dbl)
            n384 = local write "Trial Number"(w576) -> ()
            "Pert?" <- 1
          }
        }
        n385 = case shown="True" w278 {
          frame False {
            n386 = local write "Pert?"(0.0 ("Pert?")) -> ()
          }
          frame True {
            n387 = local write "TM Accel/\nDecel"(0.0 ("Step Counter")) -> ()
            n388 = local write "Left Trip"(FALSE) -> ()
            n389 = local read "Trial Number"() -> (w568:dbl)
            n390 = local write "Step Counter"(-8.0 ("Step Counter")) -> ()
            n391 = Add(x=w568, y=1.0) -> (x+y=w570:dbl)
            n392 = local write "Trial Number"(w570) -> ()
            n393 = local write "Pert?"(1.0 ("Pert?")) -> ()
          }
        }
        n394 = case shown="True" w280 {
          frame False {
            n395 = local write "Pert?"(0.0 ("Pert?")) -> ()
          }
          frame True {
            n396 = local write "TM Accel/\nDecel"(0.0 ("Step Counter")) -> ()
            n397 = local write "Right Trip"(FALSE) -> ()
            n398 = local read "Trial Number"() -> (w552:dbl)
            n399 = local write "Step Counter"(-8.0 ("Step Counter")) -> ()
            n400 = Add(x=w552, y=1.0) -> (x+y=w554:dbl)
            n401 = local write "Trial Number"(w554) -> ()
            n402 = local write "Pert?"(1.0 ("Pert?")) -> ()
          }
        }
        n403 = case shown="True" w279 {
          frame False {
            n404 = local write "Pert?"(0.0 ("Pert?")) -> ()
          }
          frame True {
            n405 = local write "TM Accel/\nDecel"(0.0 ("Step Counter")) -> ()
            n406 = local write "Right Slip"(FALSE) -> ()
            n407 = local read "Trial Number"() -> (w562:dbl)
            n408 = local write "Step Counter"(-8.0 ("Step Counter")) -> ()
            n409 = Add(x=w562, y=1.0) -> (x+y=w560:dbl)
            n410 = local write "Trial Number"(w560) -> ()
            n411 = local write "Pert?"(1.0 ("Pert?")) -> ()
          }
        }
        n412 = case shown="True" "Stop" {
          frame False {
          }
          frame True {
            n413 = local write "TM Accel/\nDecel"(0.0 ("Step Counter")) -> ()
            n414 = local write "HS Delay"(0.0 ("Step Counter")) -> ()
            n415 = local write "Perturbation\nDelay Onset"(0.0 ("Step Counter")) -> ()
            n416 = local write "Step Counter"(0.0 ("Step Counter")) -> ()
            n417 = local write "Speed Parameter"(enum32{"0.7 m/s Settings", "1.0 m/s Settings"}."0.7 m/s Settings" ("Speed Parameter")) -> ()
          }
        }
        n418 = call "Time"("Reset"="Stop") -> ("Elapsed Time (s)"=→"Elapsed Time (s)":dbl)  [unwired: 11 in, 7 out]
        n419 = node-c288() -> ()  [unwired: 1 in, 1 out]
      }
      n420 = node-c288(w238) -> ()  [unwired: 1 out]
      n421 = Close File(refnum=w216) -> ()  [unwired: 1 in, 2 out]
      n422 = TCP Close Connection(connection ID=w241, error in (no error)=w242) -> (error out=w240:errorcluster)  [unwired: 1 in, 1 out]
    }
    frame #2 {
      # "Close"
      "TM Connection" <- w849
    }
  }
